vi "Sequenced Wait.vi"(8 "Error in":errorcluster, 10 "milliseconds to wait (100)":u32=100) -> (0 "Error out":errorcluster)   [LabVIEW 2012]
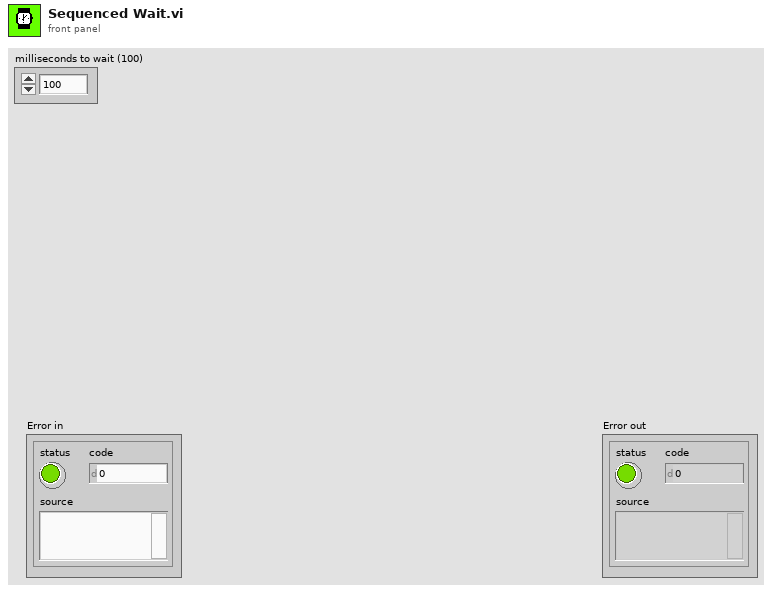
[diagram p1: front panel]
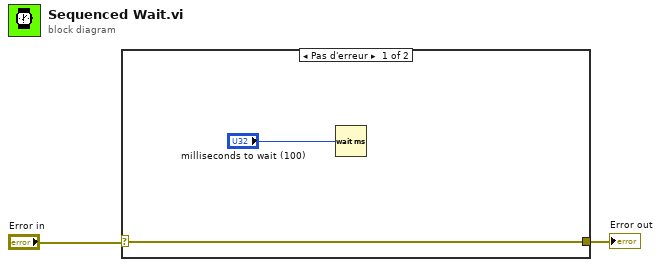
[diagram p0: block diagram]
diagram:
  n1 = case shown="Pas d'erreur" "Error in" {
    selector: "Error in" -> [w4 w5]
    tunnel: [w4 w5] -> w1
    frame No Error {
      n2 = Wait (ms)(milliseconds to wait="milliseconds to wait (100)") -> ()  [unwired: 1 out]
    }
    frame Error {
    }
  }
  "Error out" <- w1
